vi "Test Find Dashed Tests.vi"(8 "error in (no error)":errorcluster, 11 "Test Case In":refnum<class "Test FInder Test.lvclass">) -> (0 "error out":errorcluster, 3 "Test Case Out":refnum<class "Test FInder Test.lvclass">)   [LabVIEW 2020, in "Test FInder Test.lvclass"]
uses:
  Test FInder Test.lvclass
  C:/Program Files (x86)/National Instruments/LabVIEW 2020/vi.lib/Astemes/LUnit/Test Case.lvclass
  <vilib>/Astemes/LUnit/Test Case.lvclass/Test Case.ctl
  <vilib>/Astemes/LUnit/Append Fail Result.vi
  <vilib>/Astemes/LUnit/Append Pass Result.vi
  source/API/LUnit Test Suite/LUnit Test Suite.lvclass
  C:/git/astemes-lunit/source/Core/Runnable/Runnable.lvclass
  source/Framework/Test Finder/Test Finder.lvclass
  <vilib>/Astemes/LUnit/Test Case.lvclass
  source/Core/Runnable/Runnable.lvclass
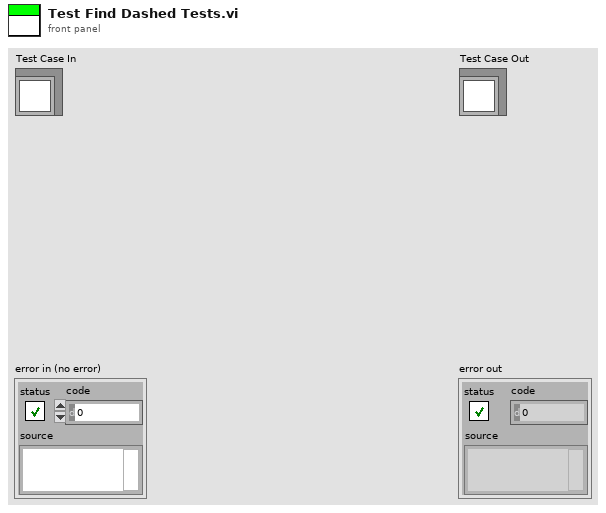
[diagram p1: front panel]
types:
  T1 = typedef "Result.lvlib/Result.ctl" = cluster{"Name":string, "Message":string, "Description":string, "Status":T2, "Result Type":T3, "Execution Time":dbl}
  T2 = typedef "Result.lvlib/Status.ctl" = enum16{"", "Passed", "Failed", "Error", "Skipped", "Setup Error", "Broken", "Teardown Error"}
  T3 = typedef "Result.lvlib/Type.ctl" = enum16{"Test Case", "Test Suite", "Test Run", "Pass", "Fail", "Skip", "Pass if", "Fail if", "Pass if Error", "Fail if Error", "Pass if Equal", "Fail if Equal"}
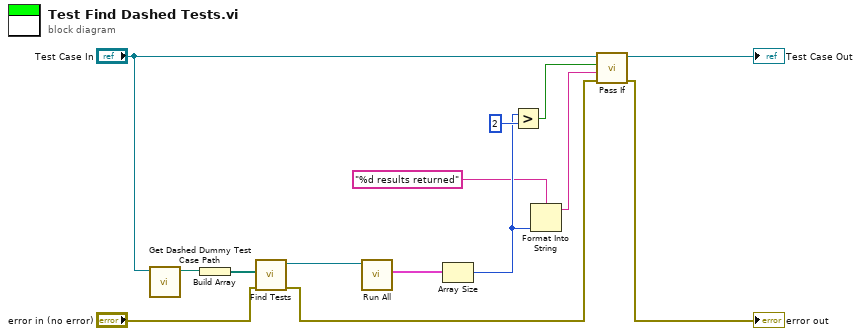
[diagram p0: block diagram]
diagram:
  n1 = call "Get Dashed Dummy Test Case Path.vi"("LUnit Test Suite Tests in"="Test Case In") -> ("appended path"=w11:path)  [unwired: 10 in]
  n2 = Build Array(w11) -> (w10:path[])
  n3 = call "Find Tests.vi"("error in (no error)"="error in (no error)", "File Paths"=w10) -> ("error out"=w12:errorcluster, "LUnit Test Suite"=w9:refnum<class "LUnit Test Suite.lvclass">)  [unwired: 8 in]
  n4 = call "Run All.vi"("Runnable In"=w9) -> ("Results"=w8:T1[])  [unwired: 9 in, 1 out]
  n5 = Array Size(array=w8) -> (size(s)=w3:i32)
  n6 = Greater?(x=w3, y=2) -> (0:w4:bool)
  n7 = Format Into String(format string="%d results returned", w3) -> (resulting string=w1:string)  [unwired: 2 in, 1 out]
  n8 = call <vilib>:"Pass If.vi"("error in (no error)"=w12, "Message"=w1, "Pass?"=w4, "LUnit Test Case In"="Test Case In") -> ("error out"=→"error out":errorcluster, "LUnit Test Case Out"=→"Test Case Out":refnum<class "Test FInder Test.lvclass">)  [unwired: 6 in]
